vi "graceful_return.vi"(8 "raster-scan-params":T1={"TsTicks"=1600, "Stop"=TRUE, "TOL"=0.3, "ramp-rate"=0.0, "z-u-max"=5.0, "PI-params"={"Ki"=0.001, "setpoint"=0.0}} {"z-u-max" format="%#_13g"; "TOL" format="%#_13g"}, 10 "uy(0)":sgl format="%#_13g", 11 "ux(0)":sgl format="%#_13g") -> ()   [LabVIEW 2015]
uses:
  raster-scan-params.ctl
  controls/PI-params.ctl
  <vilib>/rvi/Emulation/niFpgaGetClockAttributes.vi
  <vilib>/rvi/Emulation/niFpgaSctlEmulationGetInTimedLoop.vi
  <vilib>/rvi/Emulation/niFpgaEmulationReportErrorSimple.vi
  <vilib>/rvi/Emulation/niFpgaEmulationIsFPGAContextNoSignature.vi
  <vilib>/rvi/DataTransferAndStorage/Container/Common/niFpgaContainerGetUniqueNameForEmu.vi
  <vilib>/rvi/Memory/Memory_Emulation/niFpgaMemoryEmulationCacheClearOnFirstRun.vi
  <vilib>/rvi/Memory/Memory_Emulation/nirvimemoryEmulationManagerCache_MakeExclusive.vi
  <vilib>/rvi/Memory/Memory_Emulation/niFpgaMemoryEmulationValidateCache.vi
  <vilib>/rvi/Memory/Memory_Emulation/nirvimemoryEmulationManagerCache_InsertValue.vi
  <vilib>/Utility/error.llb/Clear Errors.vi
  <vilib>/rvi/Memory/Memory_Emulation/nirvimemoryEmulationManagerCache_ReleaseExclusive.vi
  <vilib>/rvi/Memory/Memory_Emulation/nirvimemoryEmulationManagerCache_GetValue.vi
  <vilib>/rvi/Memory/Memory_Emulation/nirvimemoryEmulationManagerCache_SetValue.vi
  <vilib>/rvi/Emulation/niFpgaProcessEmulError.vi
  <vilib>/rvi/eio/common/nirviEmuTemplateMethod_errors.vi
  <vilib>/rvi/Emulation/niFpgaCriticalErrorInLSC.vi
  <vilib>/rvi/DataTransferAndStorage/Container/XNode/niFpgaContainer.xnode
  <vilib>/rvi/DataTransferAndStorage/Register/Emulation/niFpgaRegisterEmulation.vi
  <vilib>/eio/EIONode/EIONode.xnode
panel:
  out "Uy":sgl
  out "Ux":sgl
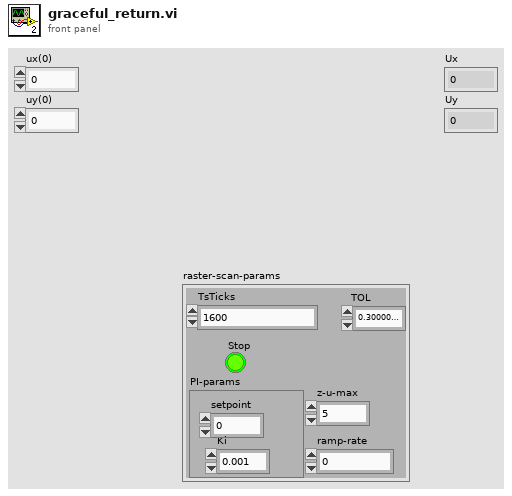
[diagram p1: front panel]
types:
  T1 = typedef "raster-scan-params.ctl" = cluster{"TsTicks":u32, "Stop":bool, "TOL":sgl, "ramp-rate":sgl, "z-u-max":sgl, "PI-params":T2}
  T2 = typedef "PI-params.ctl" = cluster{"Ki":sgl, "setpoint":sgl}
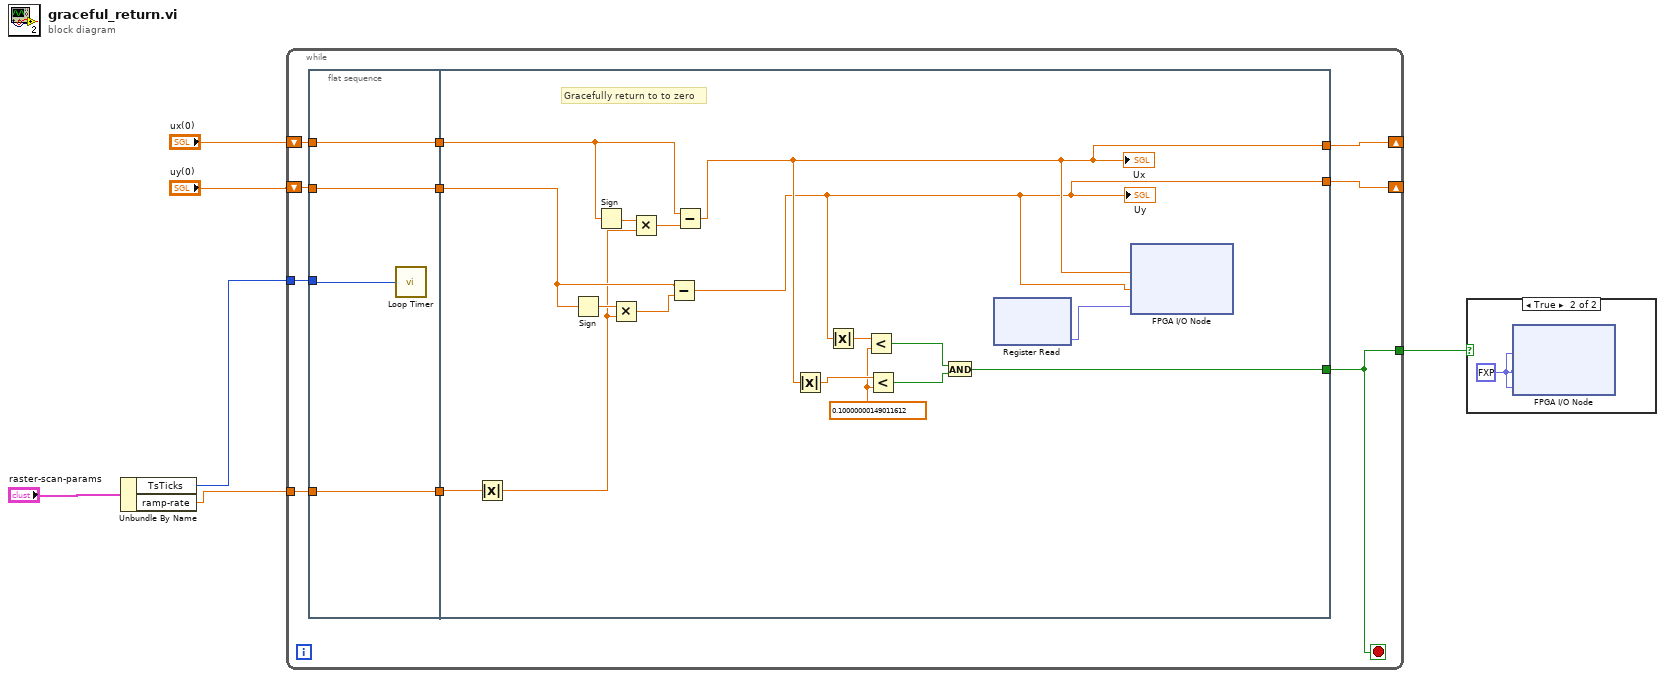
[diagram p0: block diagram]
diagram:
  n1 = Unbundle By Name("raster-scan-params") -> ("TsTicks"=w2:u32, "ramp-rate"=w1:sgl)
  n2 = while {
    tunnel: w1 -> [w13]
    shift-right: [w12] -> _
    shift-left: "uy(0)" -> [w11]
    shift-right: [w10] -> _
    shift-left: "ux(0)" -> [w9]
    tunnel: [w8] -> w4
    tunnel: w2 -> [w7]
    stop <- w8 stop-if-true
    n3 = flat-sequence {
      tunnel: [w20] -> w16
      tunnel: w11 -> [w20]
      tunnel: [w19] -> w15
      tunnel: w9 -> [w19]
      tunnel: [w18] -> w14
      tunnel: w13 -> [w18]
      tunnel: w7 -> [w17]
      tunnel: w16 -> [w27]
      tunnel: w15 -> [w28]
      tunnel: w14 -> [w22]
      tunnel: [w26] -> w8
      tunnel: [w24] -> w12
      tunnel: [w25] -> w10
      frame #0 {
        n4 = call "Loop Timer"("Count(Ticks)"=w17) -> ()  [unwired: 1 out]
      }
      frame #1 {
        w31 = sgl 0.1
        # "Gracefully return to to zero"
        n5 = Absolute Value(x=w22) -> (abs(x)=w21:sgl)
        n6 = Sign(1:w27) -> (0:w37:sgl)
        n7 = Sign(1:w28) -> (0:w34:sgl)
        n8 = Multiply(x=w37, y=w21) -> (x*y=w36:sgl)
        n9 = Multiply(x=w34, y=w21) -> (x*y=w35:sgl)
        n10 = Subtract(x=w27, y=w36) -> (x-y=w24:sgl)
        "Uy" <- w24
        n11 = Subtract(x=w28, y=w35) -> (x-y=w25:sgl)
        "Ux" <- w25
        n12 = Absolute Value(x=w25) -> (abs(x)=w32:sgl)
        n13 = Absolute Value(x=w24) -> (abs(x)=w33:sgl)
        n14 = Less?(x=w33, y=w31) -> (x < y?=w29:bool)
        n15 = Less?(x=w32, y=w31) -> (x < y?=w30:bool)
        n16 = And(x=w29, y=w30) -> (x .and. y?=w26:bool)
        n17 = xnode ("Register Read")() -> ("Data"=w23:fxp<+/-,16,5>)  [unwired: 1 in, 1 out]
        n18 = xnode "FPGA I/O Node"("Mod1/AO0"=w25, "Mod1/AO1"=w24, "Mod1/AO2"=w23) -> ()  [unwired: 3 in, 3 out]
      }
    }
  }
  n19 = case shown="True" w4 {
    frame False {
    }
    frame True {
      w38 = fxp<+,1,1> 0.0
      n20 = xnode "FPGA I/O Node"("Mod1/AO0"=w38, "Mod1/AO1"=w38, "Mod1/AO2"=w38) -> ()  [unwired: 3 in, 3 out]
    }
  }
